vi "AutoDetector_ValidatePeak.vi"(8 "Error In":errorcluster, 11 "Auto-DV Info In":T1={"Run Optimization Proc"=TRUE, "Optimization Run Bias"=3200, "Run Bias Info"=[{"Run Bias"=1600, "Peak Height"=0.0, "% Increase"=nan, "Peak Found"=FALSE}, {"Run Bias"=1700, "Peak Height"=0.0, "% Increase"=nan, "Peak Found"=FALSE}, {"Run Bias"=1800, "Peak Height"=0.0, "% Increase"=0.0, "Peak Found"=FALSE}, {"Run Bias"=1900, "Peak Height"=9180.0, "% Increase"=inf, "Peak Found"=TRUE}, {"Run Bias"=2000, "Peak Height"=1360000.0, "% Increase"=inf, "Peak Found"=TRUE}, {"Run Bias"=2100, "Peak Height"=19600000.0, "% Increase"=213407.625272, "Peak Found"=TRUE}, {"Run Bias"=2200, "Peak Height"=39400000.0, "% Increase"=2797.058824, "Peak Found"=TRUE}, {"Run Bias"=2300, "Peak Height"=47800000.0, "% Increase"=143.877551, "Peak Found"=TRUE}, {"Run Bias"=2400, "Peak Height"=52200000.0, "% Increase"=32.48731, "Peak Found"=TRUE}, {"Run Bias"=2500, "Peak Height"=53400000.0, "% Increase"=11.715481, "Peak Found"=TRUE}, {"Run Bias"=2600, "Peak Height"=53500000.0, "% Increase"=2.490421, "Peak Found"=TRUE}, {"Run Bias"=2700, "Peak Height"=53300000.0, "% Increase"=-0.187266, "Peak Found"=TRUE}, {"Run Bias"=2800, "Peak Height"=53900000.0, "% Increase"=0.747664, "Peak Found"=TRUE}, {"Run Bias"=2900, "Peak Height"=54800000.0, "% Increase"=2.814259, "Peak Found"=TRUE}, {"Run Bias"=3000, "Peak Height"=55000000.0, "% Increase"=2.040816, "Peak Found"=TRUE}, {"Run Bias"=3100, "Peak Height"=55600000.0, "% Increase"=1.459854, "Peak Found"=TRUE}, {"Run Bias"=3200, "Peak Height"=56000000.0, "% Increase"=1.818182, "Peak Found"=TRUE}]}) -> (0 "Error Out":errorcluster, 1 "Correct Run Bias Reached":bool, 2 "Optimized DV Value":u32, 3 "Auto-DV Info Out":T1)   [LabVIEW 2015]
uses:
  Controls/Auto-Detector Bias Info.ctl
  Controls/Auto-Detector Peak Info.ctl
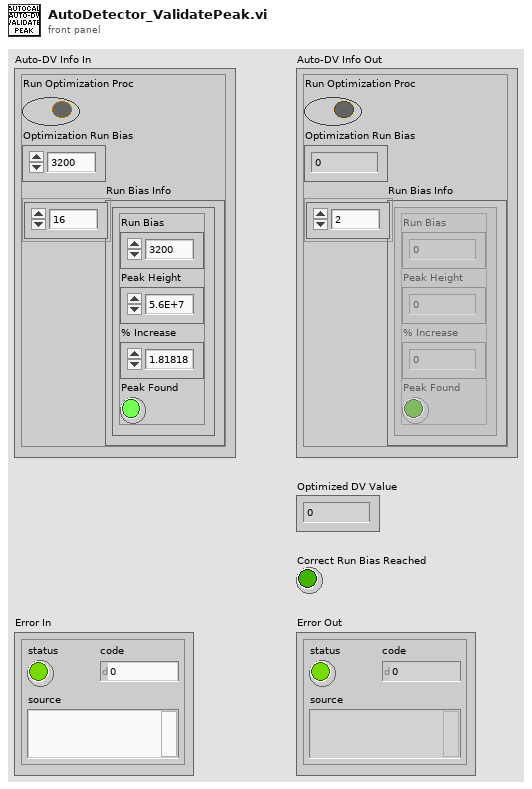
[diagram p1: front panel]
types:
  T1 = typedef "Auto-Detector Bias Info.ctl" = cluster{"Run Optimization Proc":bool, "Optimization Run Bias":u32, "Run Bias Info":T2[]}
  T2 = typedef "Auto-Detector Peak Info.ctl" = cluster{"Run Bias":u32, "Peak Height":dbl, "% Increase":dbl, "Peak Found":bool}
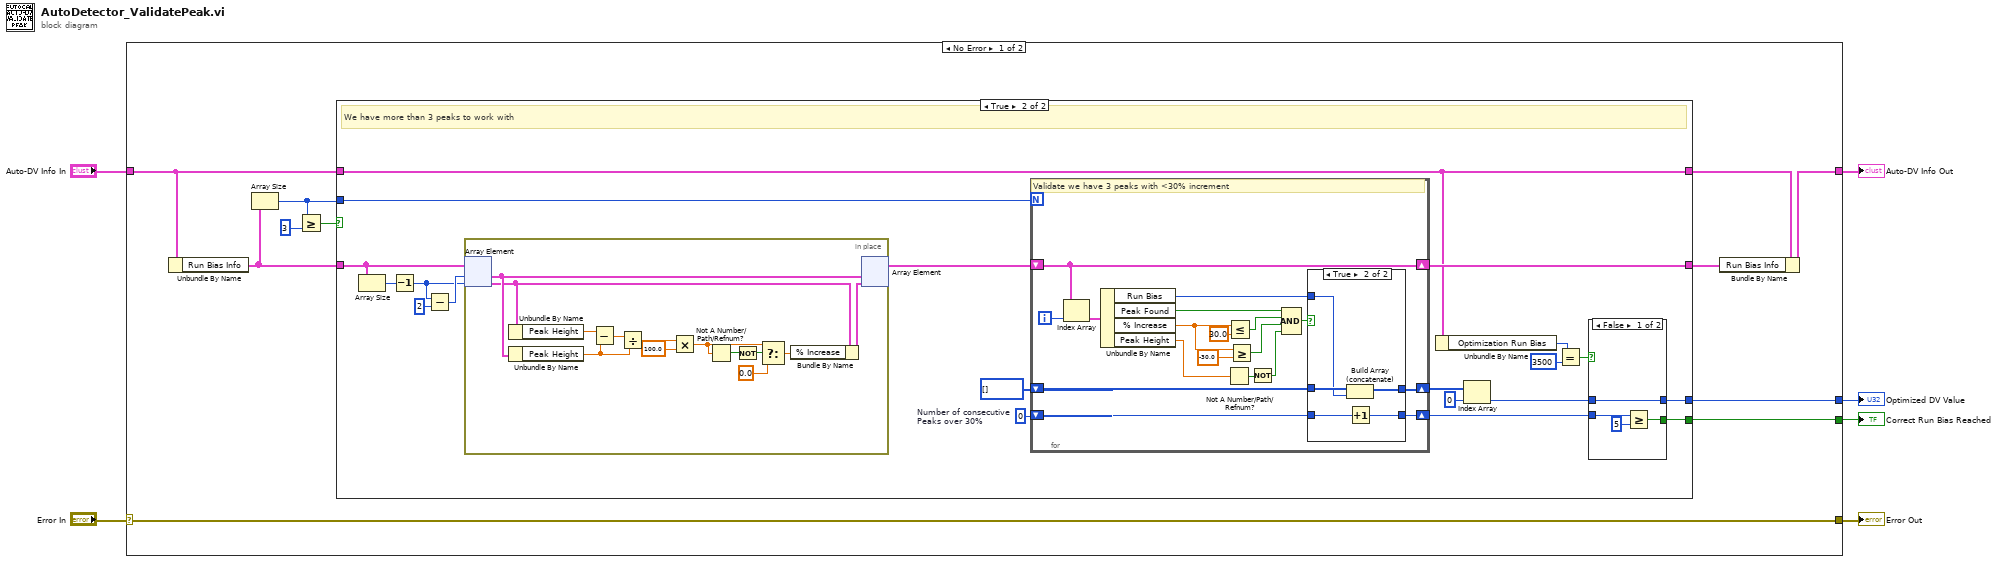
[diagram p0: block diagram]
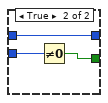
[diagram p3: hidden frame]
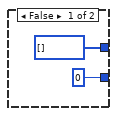
[diagram p4: hidden frame]
diagram:
  n1 = case shown="No Error" "Error In" {
    selector: "Error In" -> [w17 w86]
    tunnel: [w17 w86] -> w5
    tunnel: "Auto-DV Info In" -> [w16 w85]
    tunnel: [w15 w85] -> w3
    tunnel: [w14 _] -> w2
    tunnel: [w13 _] -> w1
    frame No Error {
      n2 = Unbundle By Name(w16) -> ("Run Bias Info"=w9:T2[])
      n3 = Array Size(array=w9) -> (size(s)=w8:i32)
      n4 = Greater Or Equal?(x=w8, y=3) -> (x >= y?=w11:bool)
      n5 = case shown="True" w11 {
        tunnel: w16 -> [w19 w31]
        tunnel: [w19 w31] -> w10
        tunnel: w9 -> [w18 w39]
        tunnel: w8 -> [_ w37]
        tunnel: [w18 w32] -> w7
        tunnel: [_ w27] -> w14
        tunnel: [_ w24] -> w13
        frame False {
          # "Not enough peaks"
        }
        frame True {
          w36 = 0  # Number of consecutive Peaks over 30%
          # "We have more than 3 peaks to work with"
          n6 = Array Size(array=w39) -> (size(s)=w23:i32)
          n7 = Decrement(x=w23) -> (x-1=w20:i32)
          n8 = Subtract(x=w20, y=2) -> (x-y=w21:i32)
          n9 = in-place {
            n10 = in-place-array #1(w39, w21, w20) -> (w83:T2, w82:T2)
            n11 = Unbundle By Name(w82) -> ("Peak Height"=w81:dbl)
            n12 = Unbundle By Name(w83) -> ("Peak Height"=w79:dbl)
            n13 = Subtract(x=w81, y=w79) -> (x-y=w80:dbl)
            n14 = Divide(x=w80, y=w79) -> (x/y=w78:dbl)
            n15 = Multiply(x=w78, y=100.0) -> (x*y=w77:dbl)
            n16 = Not A Number/Path/Refnum?(number/path/refnum=w77) -> (NaN/Path/Refnum?=w75:bool)
            n17 = Not(x=w75) -> (.not. x?=w74:bool)
            n18 = Select(t=w77, s=w74, f=0.0) -> (s? t:f=w72:dbl)
            n19 = Bundle By Name(cluster=w82, "% Increase"=w72) -> (w84:T2)
            n20 = in-place-array #1(w83, w84) -> (w38:T2[])  [unwired: 2 out]
          }
          n21 = for {
            N: w37 -> [_]
            shift-right: [w64] -> w32
            shift-left: w38 -> [w64]
            shift-right: [w60] -> w25
            shift-left: w36 -> [w59]
            shift-right: [w56] -> w34
            shift-left: u32[] [] ("Run Bias") -> [w57]
            i -> [w63]
            # "Validate we have 3 peaks with <30% increment"
            n22 = Index Array(array=w64, index=w63) -> (element=w62:T2)
            n23 = Unbundle By Name(w62) -> ("Run Bias"=w58:u32, "Peak Found"=w55:bool, "% Increase"=w49:dbl, "Peak Height"=w53:dbl)
            n24 = Not A Number/Path/Refnum?(number/path/refnum=w53) -> (NaN/Path/Refnum?=w52:bool)
            n25 = Less Or Equal?(x=w49, y=30.0) -> (x <= y?=w54:bool)
            n26 = Greater Or Equal?(x=w49, y=-30.0) -> (x >= y?=w47:bool)
            n27 = Not(x=w52) -> (.not. x?=w51:bool)
            n28 = Compound Arithmetic op=AND(w55, w54, w47, w51) -> (w50:bool)
            n29 = case shown="True" w50 {
              tunnel: [0 ("Number of consecutive Peaks over 30%") w70] -> w60
              tunnel: w59 -> [_ w71]
              tunnel: w58 -> [_ w67]
              tunnel: w57 -> [_ w69]
              tunnel: [u32[] [] ("Run Bias") w68] -> w56
              frame False {
              }
              frame True {
                n30 = Build Array (concatenate)(w69, w67) -> (w68:u32[])
                n31 = Increment(x=w71) -> (x+1=w70:i32)
              }
            }
          }
          n32 = Unbundle By Name(w31) -> ("Optimization Run Bias"=w30:u32)
          n33 = Index Array(array=w34, index=0) -> (element=w28:u32)
          n34 = Equal?(x=w30, y=u32 3500) -> (x = y?=w26:bool)
          n35 = case shown="False" w26 {
            tunnel: w28 -> [w43 w46]
            tunnel: [w43 w46] -> w27
            tunnel: w25 -> [w41 w44]
            tunnel: [w40 w45] -> w24
            frame False {
              n36 = Greater Or Equal?(x=w41, y=5) -> (x >= y?=w40:bool)
            }
            frame True {
              n37 = Not Equal To 0?(x=w44) -> (x != 0?=w45:bool)
            }
          }
        }
      }
      n38 = Bundle By Name(cluster=w10, "Run Bias Info"=w7) -> (w15:T1)
    }
    frame Error {
    }
  }
  "Error Out" <- w5
  "Auto-DV Info Out" <- w3
  "Optimized DV Value" <- w2
  "Correct Run Bias Reached" <- w1
